vi "Check Obj Pos.vi"(7 "Pane Coordinates":T1, 8 "error in (no error)":errorcluster, 11 "Boolean Object Position in":refnum<class "Boolean Object Position.lvclass">) -> (0 "error out":errorcluster, 2 "Position":T2=enum."Top", 3 "Boolean Object Position out":refnum<class "Boolean Object Position.lvclass">)   [LabVIEW 2018, in "Boolean Object Position.lvclass"]
uses:
  Boolean Object Position.lvclass
  Pane Object.lvclass/Pane Position Enum.ctl
  Pane Object.lvclass/Object Coordinates.ctl
  Pane Object.lvclass/Pane Object Position.lvclass
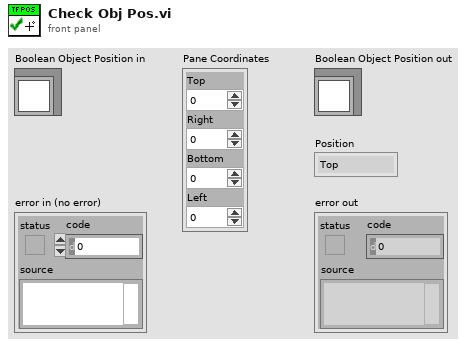
[diagram p1: front panel]
types:
  T1 = typedef "Pane Object Position.lvclass/Object Coordinates.ctl" = cluster{"Top":i32, "Right":i32, "Bottom":i32, "Left":i32}
  T2 = typedef "Pane Object Position.lvclass/Pane Position Enum.ctl" = enum16{"Indeterminate", "Top", "Right", "Top Right", "Bottom", "5", "Bottom Right", "7", "Left", "Top Left", "10", "11", "Bottom Left"}
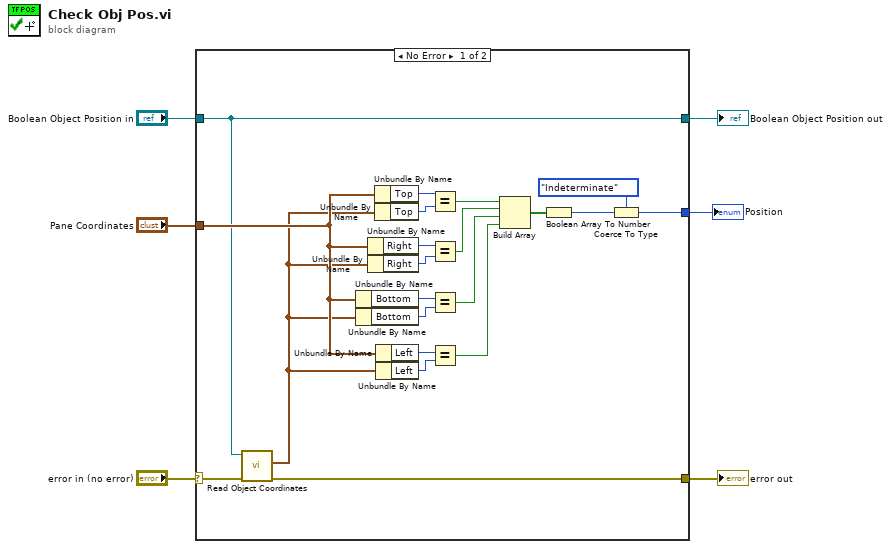
[diagram p0: block diagram]
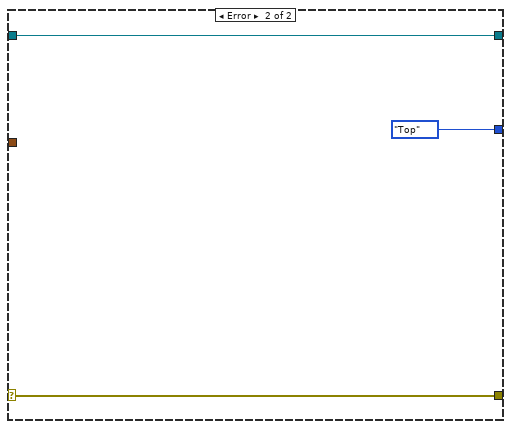
[diagram p2: hidden frame]
diagram:
  n1 = case shown="No Error" "error in (no error)" {
    selector: "error in (no error)" -> [w16 w29]
    tunnel: [w15 w29] -> w5
    tunnel: "Boolean Object Position in" -> [w18 w30]
    tunnel: [w18 w30] -> w3
    tunnel: "Pane Coordinates" -> [w19 _]
    tunnel: [w8 Pane_Position_Enum."Top" ("Position")] -> w1
    frame No Error {
      n2 = call-dynamic "Read Object Coordinates.vi"("error in (no error)"=w16, "Pane Object Position in"=w18) -> ("error out"=w15:errorcluster, "Object Coordinates"=w17:T1)  [unwired: 7 in, 1 out]
      n3 = Unbundle By Name(w19) -> ("Bottom"=w24:i32)
      n4 = Unbundle By Name(w17) -> ("Bottom"=w25:i32)
      n5 = Unbundle By Name(w19) -> ("Right"=w22:i32)
      n6 = Unbundle By Name(w17) -> ("Right"=w23:i32)
      n7 = Unbundle By Name(w19) -> ("Top"=w20:i32)
      n8 = Unbundle By Name(w17) -> ("Top"=w21:i32)
      n9 = Unbundle By Name(w19) -> ("Left"=w26:i32)
      n10 = Unbundle By Name(w17) -> ("Left"=w27:i32)
      n11 = Equal?(x=w20, y=w21) -> (x = y?=w13:bool)
      n12 = Equal?(x=w22, y=w23) -> (x = y?=w12:bool)
      n13 = Equal?(x=w24, y=w25) -> (x = y?=w11:bool)
      n14 = Equal?(x=w26, y=w27) -> (x = y?=w10:bool)
      n15 = Build Array(w13, w12, w11, w10) -> (w14:bool[])
      n16 = Boolean Array To Number(Boolean array=w14) -> (number=w7:u32)
      n17 = Coerce To Type(0:w7, 1:Pane_Position_Enum."Indeterminate" ("Position")) -> (2:w8:T2)
    }
    frame Error {
    }
  }
  "error out" <- w5
  "Boolean Object Position out" <- w3
  "Position" <- w1
